vi "reapply settings.vi"(10 "ws settings in":T1, 11 "desired settings":T1) -> (3 "ws settings out":T1)   [LabVIEW 2013]
uses:
  <resource>/Framework/Providers/ws_project_provider/common/Web Service.ctl
  <resource>/Framework/Providers/ws_project_provider/common/Web Service VI.ctl
  <resource>/Framework/Providers/ws_project_provider/common/Web Service VI Type.ctl
  <resource>/Framework/Providers/ws_project_provider/common/Web Service VI Method.ctl
  <resource>/Framework/Providers/ws_project_provider/common/Web Service VI Output Type.ctl
  <resource>/Framework/Providers/ws_project_provider/common/Web Service VI Output Format.ctl
  <resource>/Framework/Providers/ws_project_provider/common/NI Web Service Provider.lvlib
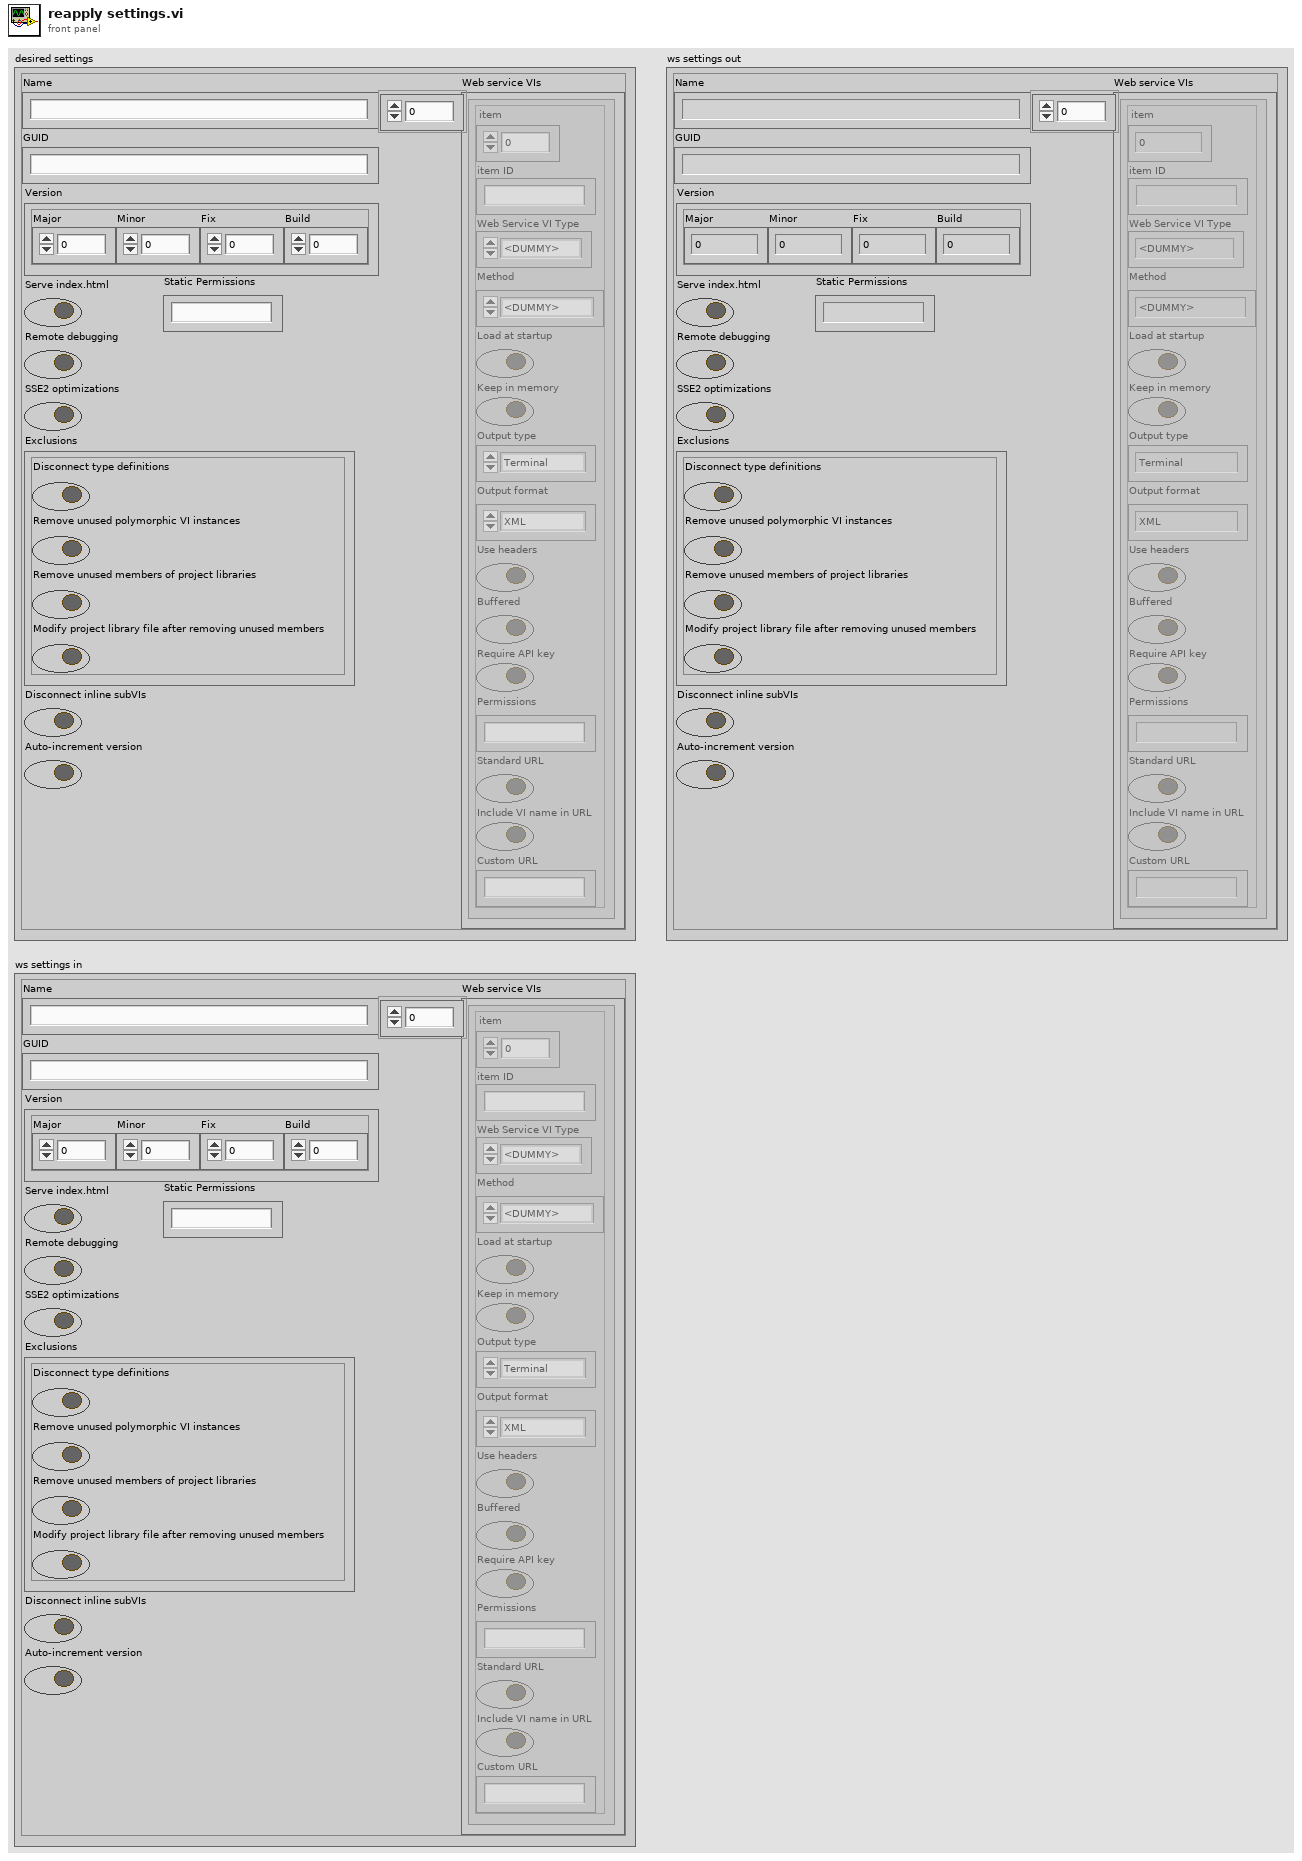
[diagram p1: front panel]
types:
  T1 = typedef "NI Web Service Provider.lvlib/Web Service.ctl" = cluster{"Name":string, "GUID":string, "Version":cluster{"Major":u16, "Minor":u16, "Fix":u16, "Build":u16}, "Serve index.html":bool, "Remote debugging":bool, "SSE2 optimizations":bool, "Exclusions":cluster{"Disconnect type definitions":bool, "Remove unused polymorphic VI instances":bool, "Remove unused members of project libraries":bool, "Modify project library file after removing unused members":bool}, "Disconnect inline subVIs":bool, "Auto-increment version":bool, "Web service VIs":T2[], "Static Permissions":string}
  T2 = typedef "NI Web Service Provider.lvlib/Web Service VI.ctl" = cluster{"item":u64, "item ID":string, "Web Service VI Type":T3, "Method":T4, "Load at startup":bool, "Keep in memory":bool, "Output type":T5, "Output format":T6, "Use headers":bool, "Buffered":bool, "Require API key":bool, "Permissions":string, "Standard URL":bool, "Include VI name in URL":bool, "Custom URL":string}
  T3 = typedef "NI Web Service Provider.lvlib/Web Service VI Type.ctl" = enum16{"<DUMMY>", "Web Method", "Auxiliary", "Internal", "Content"}
  T4 = typedef "NI Web Service Provider.lvlib/Web Service VI Method.ctl" = enum16{"<DUMMY>", "GET", "PUT", "POST", "DELETE", "OPTIONS", "HEAD", "TRACE"}
  T5 = typedef "NI Web Service Provider.lvlib/Web Service VI Output Type.ctl" = enum16{"Terminal", "Stream"}
  T6 = typedef "NI Web Service Provider.lvlib/Web Service VI Output Format.ctl" = enum16{"<DUMMY>", "Text", "XML", "HTML", "JSON"}
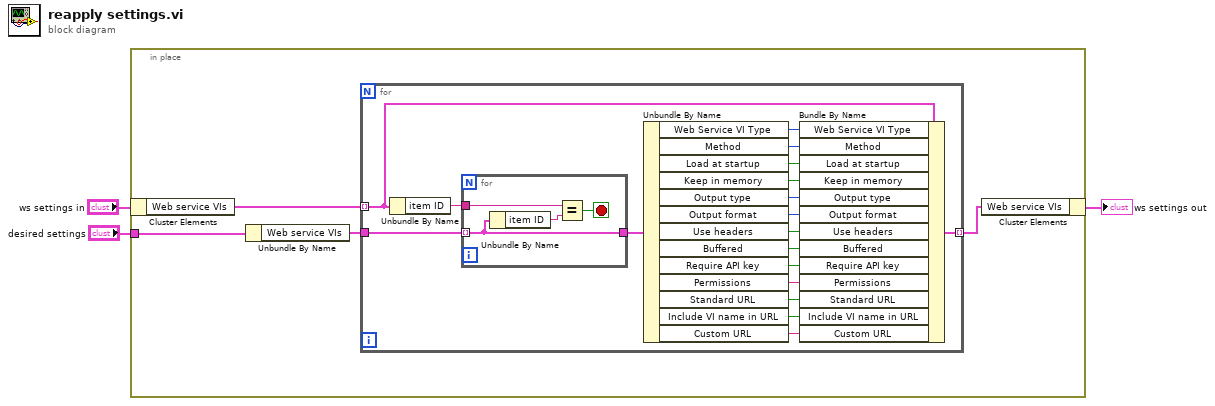
[diagram p0: block diagram]
diagram:
  n1 = in-place {
    in-place-border: "desired settings" -> [w6]
    n2 = in-place-cluster #1("ws settings in") -> ("Web service VIs"=w7:T2[])
    n3 = Unbundle By Name(w6) -> ("Web service VIs"=w5:T2[])
    n4 = for {
      tunnel: w7 -> [w22] mode=indexing
      tunnel: w5 -> [w25]
      tunnel: [w21] -> w4 mode=indexing
      n5 = Unbundle By Name(w22) -> ("item ID"=w24:string)
      n6 = for {
        tunnel: w25 -> [w27] mode=indexing
        tunnel: w24 -> [w28]
        tunnel: [w27] -> w23
        stop <- w26 stop-if-true
        n7 = Unbundle By Name(w27) -> ("item ID"=w29:string)
        n8 = Equal?(x=w28, y=w29) -> (x = y?=w26:bool)
      }
      n9 = Unbundle By Name(w23) -> ("Web Service VI Type"=w20:T3, "Method"=w19:T4, "Load at startup"=w18:bool, "Keep in memory"=w17:bool, "Output type"=w16:T5, "Output format"=w15:T6, "Use headers"=w14:bool, "Buffered"=w13:bool, "Require API key"=w12:bool, "Permissions"=w11:string, "Standard URL"=w10:bool, "Include VI name in URL"=w9:bool, "Custom URL"=w8:string)
      n10 = Bundle By Name(cluster=w22, "Web Service VI Type"=w20, "Method"=w19, "Load at startup"=w18, "Keep in memory"=w17, "Output type"=w16, "Output format"=w15, "Use headers"=w14, "Buffered"=w13, "Require API key"=w12, "Permissions"=w11, "Standard URL"=w10, "Include VI name in URL"=w9, "Custom URL"=w8) -> (w21:T2)
    }
    n11 = in-place-cluster #1("Web service VIs"=w4) -> (→"ws settings out":T1)
  }
